vi "Test image cell.vi"(11 "Test Case In":refnum<class "Test Cases.lvclass">) -> (0 "error out":errorcluster, 3 "Test Case Out":refnum<class "Test Cases.lvclass">)   [LabVIEW 2024, in "Test Cases.lvclass"]
uses:
  Test Cases.lvclass
  C:/Program Files/National Instruments/LabVIEW 2025/vi.lib/Astemes/LUnit/Test Case.lvclass
  D:/git/Sourcegrid-LabVIEW/dll/SourceGrid.dll
  dll/SourceGrid.dll
  source/Grid/SourceGrid.lvclass
  source/Cells/Image/Image.lvclass
  D:/git/Sourcegrid-LabVIEW/source/Cells/Cell/Cell.lvclass
  source/Controllers/Tool Tip Text/Tool Tip Text.lvclass
  D:/git/Sourcegrid-LabVIEW/source/Controller/IController/IController.lvclass
  <vilib>/Astemes/LUnit/Test Case.lvclass/Test Case.ctl
  <vilib>/Astemes/LUnit/Append Pass Result.vi
  <vilib>/Astemes/LUnit/Append Fail Result.vi
  <vilib>/Astemes/LUnit/Run In UI.vi
  <vilib>/Utility/error.llb/Clear Errors.vi
  source/Grid/Set Column Default Width.vi
  <vilib>/Astemes/LUnit/Test Case.lvclass
  source/Cells/Cell/Cell.lvclass
panel:
  in  "stop":bool
  in  "Grid Container":refnum<k24>(container)
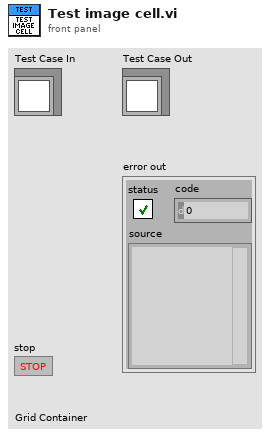
[diagram p1: front panel]
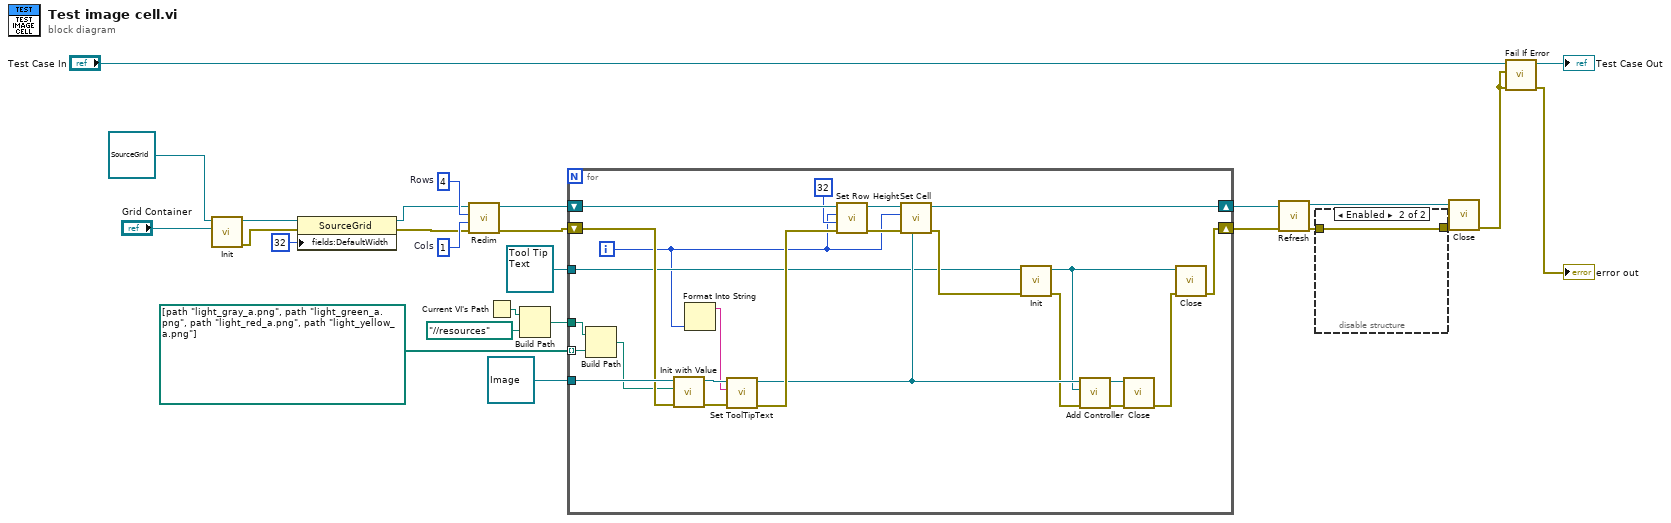
[diagram p0: block diagram]
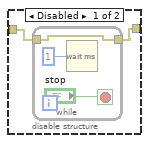
[diagram p2: hidden frame]
diagram:
  w22 = 1  # Cols
  w23 = 4  # Rows
  n1 = call-dynamic "Init.vi"("Sourcegrid Container"="Grid Container", "Grid in"=refnum<class "SourceGrid.lvclass"> refnum) -> ("error out"=w11:errorcluster, "Grid out"=w19:refnum<class "SourceGrid.lvclass">)  [unwired: 8 in]
  n2 = property class="SourceGrid"(reference=w19, error in=w11, "fields:DefaultWidth"=32 ("DefaultWidth")) -> (reference out=w18:refnum<class "SourceGrid.lvclass">, error out=w17:errorcluster)
  n3 = call "Redim.vi"("error in"=w17, "Columns"=w22, "Rows"=w23, "Sourcegrid in"=w18) -> ("error out"=w6:errorcluster, "Sourcegrid out"=w14:refnum<class "SourceGrid.lvclass">)  [unwired: 6 in]
  n4 = Current VI's Path() -> (path=w2:path)
  n5 = Build Path(base path=w2, name or relative path=path "../../resources" ("base path")) -> (appended path=w4:path)
  n6 = for {
    shift-right: [w29] -> w7
    shift-left: w6 -> [w42]
    shift-right: [w50] -> w15
    shift-left: w14 -> [w45]
    tunnel: refnum<class "Image.lvclass"> refnum ("Cell in") -> [w49]
    tunnel: path[] [path "light_gray_a.png", path "light_green_a.png", path "light_red_a.png", path "light_yellow_a.png"] -> [w47] mode=indexing
    tunnel: w4 -> [w48]
    tunnel: refnum<class "Tool Tip Text.lvclass"> refnum ("SourceGrid.lvlib:Tool Tip Text.lvclass") -> [w32]
    i -> [w28]
    n7 = Build Path(base path=w48, name or relative path=w47) -> (appended path=w41:path)
    n8 = call-dynamic "Init with Value.vi"("error in"=w42, "Value"=w41, "Image in"=w49) -> ("error out"=w46:errorcluster, "Image out"=w38:refnum<class "Image.lvclass">)  [unwired: 7 in]
    n9 = Format Into String(w28) -> (resulting string=w27:string)  [unwired: 3 in, 1 out]
    n10 = call "Set ToolTipText.vi"("error in"=w46, "ToolTipText"=w27, "Cell in"=w38) -> ("error out"=w39:errorcluster, "Cell out"=w35:refnum<class "Image.lvclass">)  [unwired: 7 in]
    n11 = call "Set Row Height.vi"("error in"=w39, "Height"=32, "Row"=w28, "SourceGrid in"=w45) -> ("error out"=w44:errorcluster, "SourceGrid out"=w43:refnum<class "SourceGrid.lvclass">)  [unwired: 6 in]
    n12 = call "Set Cell.vi"("Cell"=w35, "error in"=w44, "Row"=w28, "Sourcegrid in"=w43) -> ("error out"=w34:errorcluster, "Sourcegrid out"=w50:refnum<class "SourceGrid.lvclass">)  [unwired: 6 in]
    n13 = call-dynamic "Init.vi"("error in"=w34, "Tool Tip Text in"=w32) -> ("error out"=w33:errorcluster, "Tool Tip Text out"=w30:refnum<class "Tool Tip Text.lvclass">)  [unwired: 8 in]
    n14 = call "Add Controller.vi"("error in"=w33, "IController"=w30, "Cell in"=w35) -> ("error out"=w37:errorcluster, "Cell out"=w36:refnum<class "Image.lvclass">)  [unwired: 7 in]
    n15 = call-dynamic "Close.vi"("error in"=w37, "Cell in"=w36) -> ("error out"=w31:errorcluster)  [unwired: 8 in, 1 out]
    n16 = call-dynamic "Close.vi"("error in"=w31, "Tool Tip Text in"=w30) -> ("error out"=w29:errorcluster)  [unwired: 8 in, 1 out]
  }
  n17 = call "Refresh.vi"("error in"=w7, "SourceGrid in"=w15) -> ("error out"=w9:errorcluster, "SourceGrid out"=w12:refnum<class "SourceGrid.lvclass">)  [unwired: 8 in]
  n18 = disable-structure shown="Enabled" {
    disable-tunnel: w9 -> [w52 w56]
    disable-tunnel: [w51 w56] -> w8
    frame Disabled {
      n19 = while {
        tunnel: w52 -> [w53]
        tunnel: [w53] -> w51
        stop <- "stop" stop-if-true
        n20 = Wait (ms)(milliseconds to wait=u32 1) -> ()  [unwired: 1 out]
      }
    }
    frame Enabled {
    }
  }
  n21 = call-dynamic "Close.vi"("error in"=w8, "Sourcegrid in"=w12) -> ("error out"=w21:errorcluster)  [unwired: 8 in, 1 out]
  n22 = call <vilib>:"Fail If Error.vi"("error in (no error)"=w21, "Assert error"=w21, "LUnit Test Case In"="Test Case In") -> ("error out"=→"error out":errorcluster, "LUnit Test Case Out"=→"Test Case Out":refnum<class "Test Cases.lvclass">)  [unwired: 7 in]
